vi "Global - RT Stream Connections.vi"() -> ()   [LabVIEW 2015]
uses:
  Support VIs/Message Queue/Message Cluster.ctl
panel:
  out "Connected？":bool caption="已连接？"
  in  "RT Stream Writer":refnum<k21> caption="RT网络流写入方端点"
  in  "RT Stream Reader":refnum<k21> caption="RT网络流读取方端点"
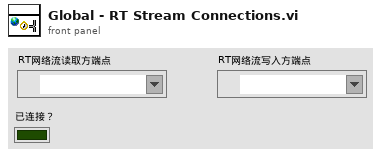
[diagram p1: front panel]
diagram:
